vi "setDAQ_Config.vi"(8 "error in (no error)":errorcluster, 10 "DAQ.Config":T1={"Channels"="", "DAQ_Type"=enum."AI", "minimum value"=-5.0, "maximum value"=5.0, "DAQ_SamplingInfo"={"Fs"=1000.0, "#s"=1000.0}, "DAQ_SamplingMode"=enum."Continuous"} {"maximum value" format="%0.2f"; "minimum value" format="%0.2f"}, 11 "DAQ in":refnum<class "DAQ.lvclass">) -> (0 "error out":errorcluster, 3 "DAQ out":refnum<class "DAQ.lvclass">)   [LabVIEW 2016, in "DAQ.lvclass"]
uses:
  DAQ.lvclass
  C:/Program Files (x86)/National Instruments/LabVIEW 2016/vi.lib/JKI/JKI SMO/SMO/SMO.lvclass
  Typedefs/DAQ_Config.ctl
  Typedefs/PrivateEvents--DAQ.AI.Channels.ctl
  Typedefs/DAQ_Type.ctl
  Typedefs/DAQ_SamplingInfo.ctl
  Typedefs/DAQ_SamplingMode.ctl
  DAQ.lvclass/DAQ.ctl
  <vilib>/JKI/JKI SMO/SMO/SMO.lvclass
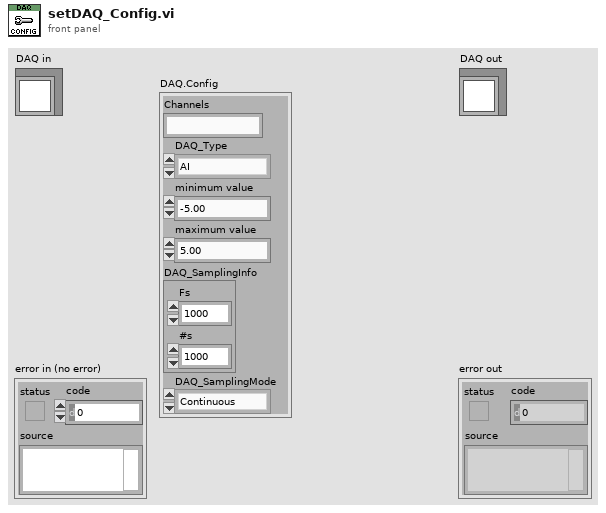
[diagram p1: front panel]
types:
  T1 = typedef "DAQ.lvclass/DAQ_Config.ctl" = cluster{"Channels":T2, "DAQ_Type":T3, "minimum value":dbl, "maximum value":dbl, "DAQ_SamplingInfo":T4, "DAQ_SamplingMode":T5}
  T2 = typedef "DAQ.lvclass/PrivateEvents--DAQ.AI.Channels.ctl" = string
  T3 = typedef "DAQ.lvclass/DAQ_Type.ctl" = enum16{"AI", "AO"}
  T4 = typedef "DAQ.lvclass/DAQ_SamplingInfo.ctl" = cluster{"Fs":dbl, "#s":dbl}
  T5 = typedef "DAQ.lvclass/DAQ_SamplingMode.ctl" = enum16{"Continuous", "Finite"}
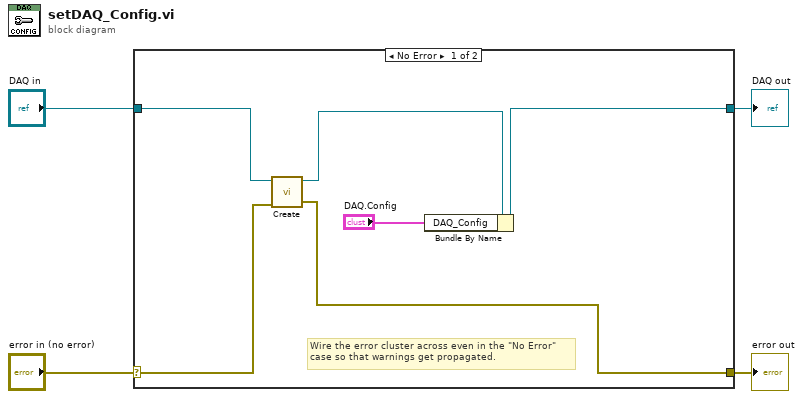
[diagram p0: block diagram]
diagram:
  n1 = case shown="No Error" "error in (no error)" {
    selector: "error in (no error)" -> [w9 w12]
    tunnel: [w6 w12] -> w3
    tunnel: [w5 w11] -> w1
    tunnel: "DAQ in" -> [w10 w11]
    frame No Error {
      # "Wire the error cluster across even in the \"No Error\"\ncase so that warnings get propagated."
      n2 = call <vilib>:"Create.vi"("error in (no error)"=w9, "SMO"=w10) -> ("error out"=w6:errorcluster, "SMO out"=w8:refnum<class "DAQ.lvclass">)  [unwired: 7 in, 1 out]
      n3 = Bundle By Name(cluster=w8, "DAQ_Config"="DAQ.Config") -> (w5:refnum<class "DAQ.lvclass">)
    }
    frame Error {
    }
  }
  "error out" <- w3
  "DAQ out" <- w1
